vi "Send Macro Exit to All Modules.vi"(8 "error in (no error)":errorcluster) -> (0 "error out":errorcluster)   [LabVIEW 2020]
uses:
  <userlib>/_NEVSTOP/Communicable State Machine(CSM)/Communicable State Machine.lvlib
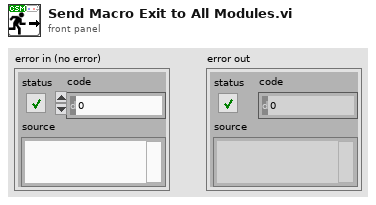
[diagram p1: front panel]
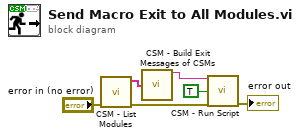
[diagram p0: block diagram]
diagram:
  n1 = call <userlib>:"CSM - List Modules.vi"("Error In"="error in (no error)") -> ("error out"=w4:errorcluster, "Module Names"=w1:string[])  [unwired: 9 in]
  n2 = call <userlib>:"CSM - Build Exit Messages of CSMs.vi"("CSMs"=w1) -> ("States"=w2:string)  [unwired: 14 in]
  n3 = call <userlib>:"CSM - Run Script.vi"("CSM Scripts"=w2, "Continue If Error? (F)"=TRUE, "error in (no error)"=w4) -> ("error out"=→"error out":errorcluster)  [unwired: 10 in, 2 out]
